vi "PTSequencer.clear list.vi"(0 "i ref in":refnum<vi>, 3 "ms timeout (10000)":i32=10000, 5 "error in (no error)":errorcluster) -> (14 "i ref out":refnum<vi>, 17 "timed out":bool, 19 "error out":errorcluster)   [LabVIEW 2014, in "PTSequencer.lvlib"]
uses:
  PTSequencer.lvlib
  CSCore/CSSystem/CSSystemLib/CSSystemLib.lvlib
  _common/PTUtils/PTUtils.lvlib
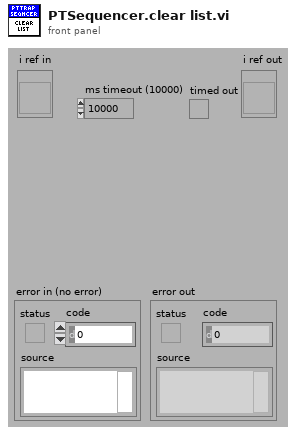
[diagram p1: front panel]
types:
  T1 = typedef "PTSequencer.lvlib/PTSequencer.i attribute.ctl" = cluster{"subsequence":bool, "mode":T2, "i step":i32, "nofLoops":i32, "i loop":i32, "Running":bool, "Paused":bool, "step done":bool, "loop done":bool, "seq done":bool, "DIM IDs":cluster{"step done":i32, "loop done":i32, "seq done":i32, "i step":i32, "i loop":i32}, "use stop conditions":bool, "stop conditions":T3[], "Step List":T5[], "DIM subsriptions":string[], "stop cond indexes":i32[], "step cond indexes":cluster{"step condition IDs":cluster{"step ID":i32, "condition ID":i32}[]}[], "Delay Start Time":timestamp, "status":string, "stopping":bool}
  T2 = typedef "PTSequencer.lvlib/PTSequencer.mode.ctl" = enum16{"single", "loop", "for loop"}
  T3 = typedef "PTSequencer.lvlib/PTSequencer.DIM service condition.ctl" = cluster{"DIM service":string, "descr":string, "nomValue":T4, "actValue":T4, "matched":bool, "DIM Status":cluster{"no link":bool, "quality":i32, "Time Stamp":timestamp}}
  T4 = typedef "CoreDefs.rawDataType.ctl" = i8[]
  T5 = typedef "PTSequencer.lvlib/PTSequencer.step.ctl" = cluster{"description":string, "object parameters":cluster{"object":string, "selector":string, "descriptor":string, "data":T4, "subsequence":bool, "call mode":enum16{"Simple DIM", "Synchronous"}, "data in":T4}, "result action":cluster{"check":bool, "passed":enum16{"Next", "Previous", "Repeat", "Jump"}, "failed":enum16{"Next", "Previous", "Repeat", "Jump"}, "jumpID_passed":i32, "jumpID_failed":i32}, "conditions":T3[], "fulfilled ":bool, "use delay":bool, "delay time (s)":dbl, "ID":i32}
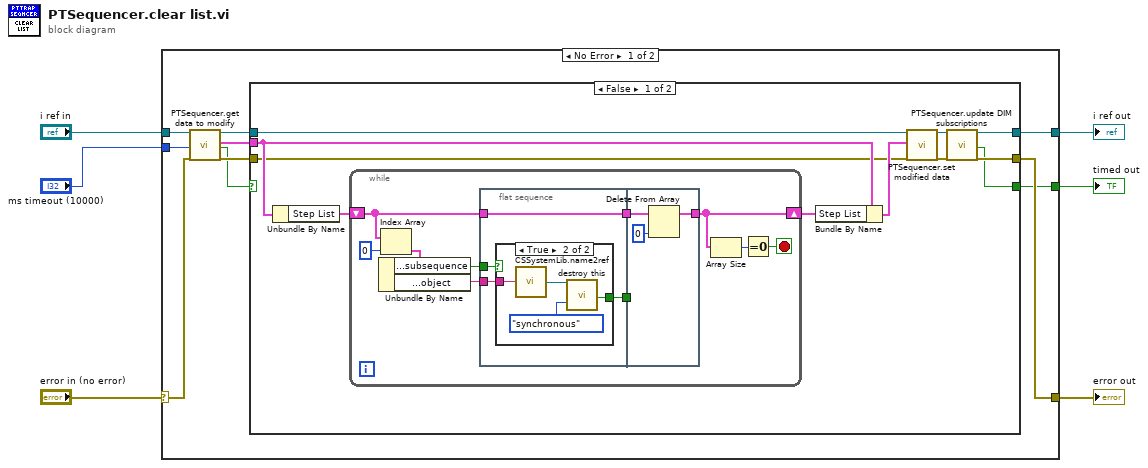
[diagram p0: block diagram]
diagram:
  n1 = case shown="No Error" "error in (no error)" {
    selector: "error in (no error)" -> [w13 w52]
    tunnel: "i ref in" -> [w16 w53]
    tunnel: [w8 w53] -> w5
    tunnel: "ms timeout (10000)" -> [w10 _]
    tunnel: [w7 _] -> w2
    tunnel: [w9 w52] -> w1
    frame No Error {
      n2 = call "PTSequencer.get data to modify.vi"("i ref in"=w16, "ms timeout (10000)"=w10, "error in (no error)"=w13) -> ("i ref out"=w15:refnum<vi>, "i attribute"=w14:T1, "timed out"=w11:bool, "error out"=w12:errorcluster)  [unwired: 13 in]
      n3 = case shown="False" w11 {
        selector: w11 -> [_ w49]
        tunnel: w15 -> [w27 w50]
        tunnel: [w22 w50] -> w8
        tunnel: w14 -> [w25 _]
        tunnel: w12 -> [w24 w51]
        tunnel: [w21 w51] -> w9
        tunnel: [w19 w49] -> w7
        frame False {
          n4 = Unbundle By Name(w25) -> ("Step List"=w18:T5[])
          n5 = while {
            shift-right: [w31] -> w17
            shift-left: w18 -> [w34]
            stop <- w29 stop-if-true
            n6 = Index Array(array=w34, index=0) -> (element=w33:T5)
            n7 = Unbundle By Name(w33) -> ("object parameters.subsequence"=w36:bool, "object parameters.object"=w35:string)
            n8 = flat-sequence {
              tunnel: w36 -> [w41]
              tunnel: w35 -> [w40]
              tunnel: w34 -> [w39]
              tunnel: [w39] -> w37
              tunnel: [w38] -> w28
              tunnel: w37 -> [w48]
              tunnel: [w47] -> w31
              tunnel: w28 -> [_]
              frame #0 {
                n9 = case shown="True" w41 {
                  tunnel: w40 -> [_ w45]
                  tunnel: [_ w42] -> w38
                  frame False {
                  }
                  frame True {
                    n10 = call "CSSystemLib.name2ref.vi"("name"=w45) -> ("obj refnum"=w44:refnum<vi>)
                    n11 = call "destroy this.vi"("i ref in"=w44, "CallType"=enum16{"simple", "synchronous", "asynchronous"}."synchronous") -> ("obj destroyed"=w42:bool)  [unwired: 17 in]
                  }
                }
              }
              frame #1 {
                n12 = Delete From Array(array=w48, index=0) -> (array with subset deleted=w47:T5[])  [unwired: 1 in, 1 out]
              }
            }
            n13 = Array Size(array=w31) -> (size(s)=w30:i32)
            n14 = Equal To 0?(x=w30) -> (x = 0?=w29:bool)
          }
          n15 = Bundle By Name(cluster=w25, "Step List"=w17) -> (w26:T1)
          n16 = call "PTSequencer.set modified data.vi"("i ref in"=w27, "CLASS.i attribute"=w26, "error in (no error)"=w24) -> ("i ref out"=w23:refnum<vi>, "error out"=w20:errorcluster)  [unwired: 15 in]
          n17 = call "PTSequencer.update DIM subscriptions.vi"("i ref in"=w23, "error in"=w20) -> ("i ref out"=w22:refnum<vi>, "timed out"=w19:bool, "error out"=w21:errorcluster)  [unwired: 15 in]
        }
        frame True {
        }
      }
    }
    frame Error {
    }
  }
  "error out" <- w1
  "i ref out" <- w5
  "timed out" <- w2
